vi "Get Method Flags.vi"(8 "error in (no error)":errorcluster, 10 "Method ID":string="36", 11 "Class ID":string="36") -> (0 "error out":errorcluster, 3 "Method Flags":T1)   [LabVIEW 2023]
doc: "<b> </b> <b> </b>\n© 2017 Q Software Innovations, LLC\nwritten by Quentin \"Q\" Alldredge\nproduced in LabVIEW 2015\n\nsupport@qsoftwareinnovations.com\nwww.qsoftwareinnovations.com\n\nAll rights reserved.\n\nRedistribution and use in source and binary forms, with or without modification, are permitted provided that the following conditions are met:\n\n * Redistributions of source code must retain the above copyright notice, this list of conditions and the following disclaimer.\n * Redistributions in binary form must reproduce the above copyright notice, this list of conditions and the following disclaimer in the documentation and/or other materials provided with the distribution.\n * Neither the name of Q Software Innovations, LLC. nor the names of its contributors may be used to endorse or promote products derived from this software without specific prior written permission.\n\nTHIS SOFTWARE IS PROVIDED BY THE COPYRIGHT HOLDERS AND CONTRIBUTORS \"AS IS\" AND ANY EXPRESS OR IMPLIED WARRANTIES, INCLUDING, BUT NOT LIMITED TO, THE IMPLIED WARRANTIES OF MERCHANTABILITY AND FITNESS FOR A PARTICULAR PURPOSE ARE DISCLAIMED. IN NO EVENT SHALL THE COPYRIGHT OWNER OR CONTRIBUTORS BE LIABLE FOR ANY DIRECT, INDIRECT, INCIDENTAL, SPECIAL, EXEMPLARY, OR CONSEQUENTIAL DAMAGES (INCLUDING, BUT NOT LIMITED TO, PROCUREMENT OF SUBSTITUTE GOODS OR SERVICES; LOSS OF USE, DATA, OR PROFITS; OR BUSINESS INTERRUPTION) HOWEVER CAUSED AND ON ANY THEORY OF LIABILITY, WHETHER IN CONTRACT, STRICT LIABILITY, OR TORT (INCLUDING NEGLIGENCE OR OTHERWISE) ARISING IN ANY WAY OUT OF THE USE OF THIS SOFTWARE, EVEN IF ADVISED OF THE POSSIBILITY OF SUCH DAMAGE."
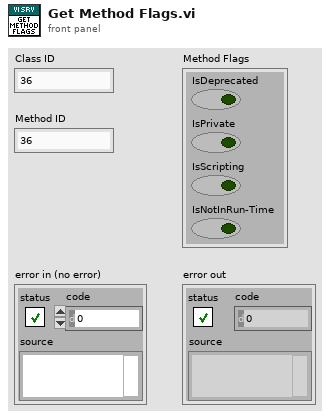
[diagram p1: front panel]
types:
  T1 = cluster{"IsDeprecated":bool, "IsPrivate":bool, "IsScripting":bool, "IsNotInRun-Time":bool}
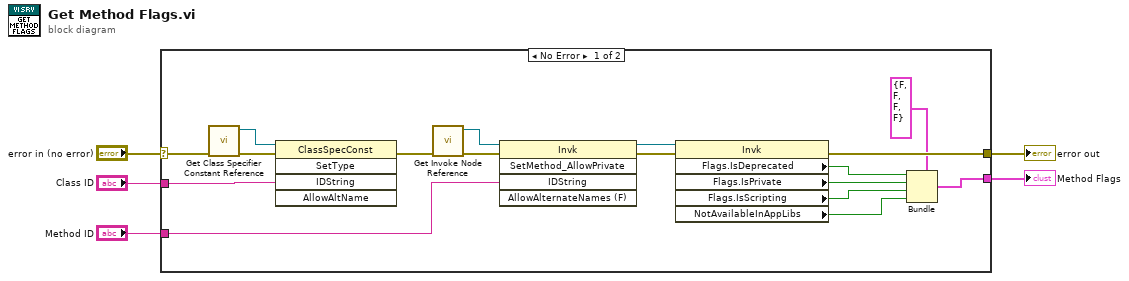
[diagram p0: block diagram]
diagram:
  n1 = case shown="No Error" "error in (no error)" {
    selector: "error in (no error)" -> [w22 w23]
    tunnel: [w15 w23] -> w4
    tunnel: "Class ID" -> [w19 _]
    tunnel: "Method ID" -> [w8 _]
    tunnel: [w13 _] -> w1
    frame No Error {
      n2 = call "Get Class Specifier Constant Reference.vi"("error in (no error)"=w22) -> ("error out"=w20:errorcluster, "specific class reference"=w21:refnum<vi>)  [unwired: 9 in]
      n3 = invoke class="ClassSpecConst" method="SetType"(reference=w21, error in=w20, "IDString"=w19) -> (error out=w18:errorcluster)  [unwired: 2 in, 4 out]
      n4 = call "Get Invoke Node Reference.vi"("error in (no error)"=w18) -> ("error out"=w17:errorcluster, "Invoke Refnum"=w16:refnum<vi>)  [unwired: 9 in]
      n5 = invoke class="Invk" method="SetMethod_AllowPrivate"(reference=w16, error in=w17, "IDString"=w8) -> (reference out=w6:refnum<vi>, error out=w7:errorcluster)  [unwired: 2 in, 3 out]
      n6 = property class="Invk"(reference=w6, error in=w7) -> (error out=w15:errorcluster, "Flags.IsDeprecated"=w10:bool, "Flags.IsPrivate"=w11:bool, "Flags.IsScripting"=w12:bool, "NotAvailableInAppLibs"=w9:bool)  [unwired: 1 out]
      n7 = Bundle(cluster=T1 {"IsDeprecated"=FALSE, "IsPrivate"=FALSE, "IsScripting"=FALSE, "IsNotInRun-Time"=FALSE}, "IsDeprecated"=w10, "IsPrivate"=w11, "IsScripting"=w12, "IsNotInRun-Time"=w9) -> (w13:T1)
    }
    frame Error {
    }
  }
  "error out" <- w4
  "Method Flags" <- w1
